vi "ORS_timestamp.vi"() -> (0 "system time":string)   [LabVIEW 2024]
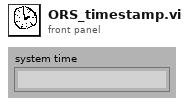
[diagram p1: front panel]
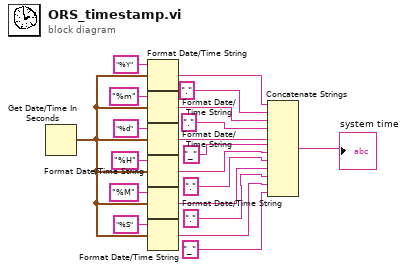
[diagram p0: block diagram]
diagram:
  n1 = Get Date/Time In Seconds() -> (seconds since 1Jan1904=w20:timestamp)
  n2 = Format Date/Time String(time format string (%c)="%Y", seconds (now)=w20) -> (date/time string=w13:string)  [unwired: 1 in]
  n3 = Format Date/Time String(time format string (%c)="%m", seconds (now)=w20) -> (date/time string=w11:string)  [unwired: 1 in]
  n4 = Format Date/Time String(time format string (%c)="%d", seconds (now)=w20) -> (date/time string=w9:string)  [unwired: 1 in]
  n5 = Format Date/Time String(time format string (%c)="%H", seconds (now)=w20) -> (date/time string=w7:string)  [unwired: 1 in]
  n6 = Format Date/Time String(time format string (%c)="%M", seconds (now)=w20) -> (date/time string=w5:string)  [unwired: 1 in]
  n7 = Format Date/Time String(time format string (%c)="%S", seconds (now)=w20) -> (date/time string=w3:string)  [unwired: 1 in]
  n8 = Concatenate Strings(w13, ".", w11, ".", w9, "_", w7, ".", w5, ".", w3, "_") -> (→"system time":string)
